vi "Write Active Cameras.vi"(8 "error in (no error)":errorcluster, 10 "Active Cameras":T1[](array[typedef]), 11 "Viewer in":refnum<class "Viewer.lvclass">) -> (0 "error out":errorcluster, 3 "Viewer out":refnum<class "Viewer.lvclass">)   [LabVIEW 2015, in "Viewer.lvlib" / "Viewer.lvclass"]
uses:
  Viewer.lvclass
  Resources/Type Defs/Camera Type.ctl
  Resources/Type Defs/Physical Camera Assignment.ctl
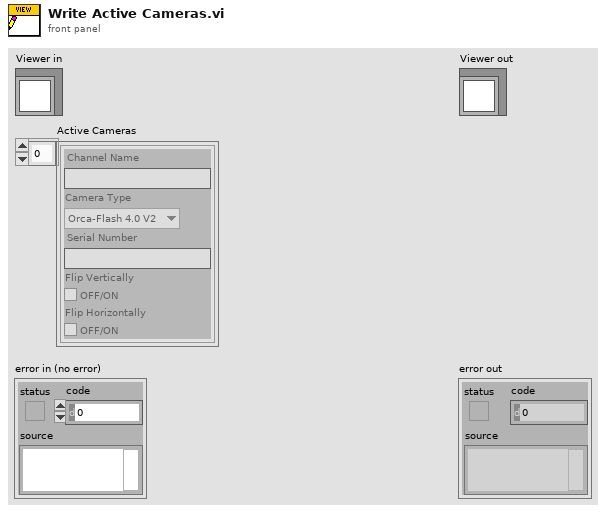
[diagram p1: front panel]
types:
  T1 = typedef "Physical Camera Assignment.ctl" = cluster{"Channel Name":string, "Camera Type":T2, "Serial Number":string, "Flip Vertically":bool, "Flip Horizontally":bool}
  T2 = typedef "Camera Type.ctl" = enum16{"Orca-Flash 4.0 V2"}
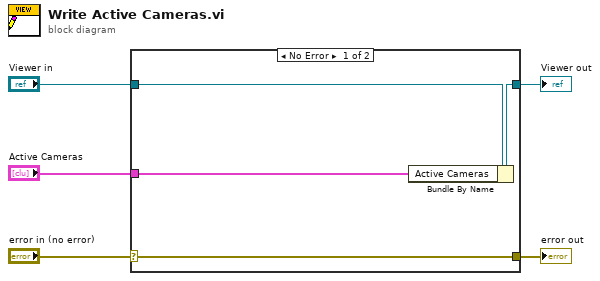
[diagram p0: block diagram]
diagram:
  n1 = case shown="No Error" "error in (no error)" {
    selector: "error in (no error)" -> [w9 w10]
    tunnel: [w9 w10] -> w4
    tunnel: [w7 w11] -> w2
    tunnel: "Viewer in" -> [w8 w11]
    tunnel: "Active Cameras" -> [w6 _]
    frame No Error {
      n2 = Bundle By Name(cluster=w8, "Active Cameras"=w6) -> (w7:refnum<class "Viewer.lvclass">)
    }
    frame Error {
    }
  }
  "error out" <- w4
  "Viewer out" <- w2
